vi "GET_1BIT_Command.vi"(9 "Canal":u8, 10 "Marca":T1) -> (1 "length":i32, 2 "Expected Response":string, 3 "Command":string, 4 "Bytes Expected":u32=2)   [LabVIEW 2019, in "Serial Device.lvclass"]
doc: "This Vi Generates the command of Read 1 Bit for each microcontroller"
uses:
  Serial Device.lvclass
  Marca.ctl
  Comando.ctl
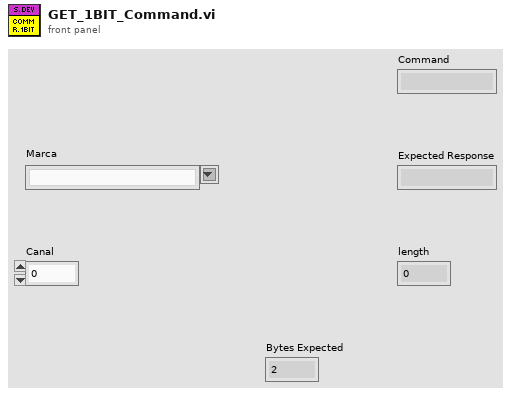
[diagram p1: front panel]
types:
  T1 = typedef "Marca.ctl" = string
  T2 = typedef "Comando.ctl" = string
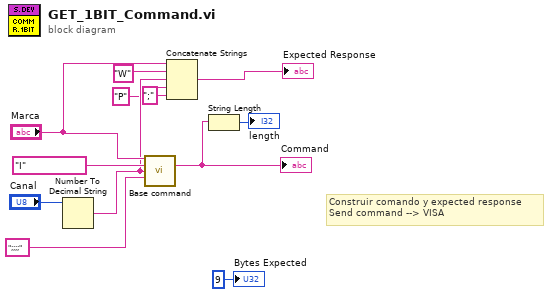
[diagram p0: block diagram]
diagram:
  # "Construir comando y expected response\nSend command --> VISA"
  n1 = Number To Decimal String(number="Canal") -> (decimal integer string=w3:string)  [unwired: 1 in]
  n2 = call "Base command.vi"("Marca"="Marca", "Comando"=T2 "I", "Parametro 1"=w3, "Parametro 2"=";;;;") -> ("Command"=w9:string)  [unwired: 10 in, 1 out]
  "Command" <- w9
  n3 = Concatenate Strings("Marca", "W", w3, "P", ";" ("string")) -> (→"Expected Response":string)
  n4 = String Length(string=w9) -> (length=→"length":i32)
  "Bytes Expected" <- u32 9 ("byte count")
